vi "Data_Acquisition(I&O).vi"(7 "Cluster":T1={"valve1Switch"=FALSE, "valve2Switch"=FALSE, "valve3Switch"=FALSE, "valve4Switch"=TRUE, "valve5Switch"=FALSE, "valve6Switch"=TRUE} caption="簇") -> ()   [LabVIEW 2020]
uses:
  <vilib>/Platform/TimedLoop/XDataNode/XDataNode.xnode
  <vilib>/Platform/TimedLoop/XDataNode/nitl_modes.ctl
  <vilib>/Platform/TimedLoop/XDataNode/XDNodeRunTimeDep.lvlib
  <vilib>/Platform/TimedLoop/XDataNode/wakeup.ctl
  <vilib>/Platform/TimedLoop/XDataNode/timing_clust.ctl
  <vilib>/rvi/interface/nirviOpenFPGA/nirviOpenFPGA.xnode
  <vilib>/rvi/interface/nirviReadWriteControl/nirviReadWriteControl.xnode
  <vilib>/rvi/interface/nirviMethod/nirviMethod.xnode
  <vilib>/FPGAPlugInAG/Dynamic/niLvFpga_Download_Dynamic.vi
  <vilib>/FPGAPlugInAG/Dynamic/niLvFpga_Reset_Dynamic.vi
  <vilib>/FPGAPlugInAG/Dynamic/niLvFpga_Run_Dynamic.vi
  <vilib>/rvi/interface/nirviCloseFPGA/nirviCloseFPGA.xnode
  <vilib>/rvi/interface/Simulation/niFpgaSimulationCallBeginRW.vi
  <vilib>/rvi/errors/niLvFpgaAdjustHostInterfaceError.vi
  <vilib>/Utility/error.llb/Error Cluster From Error Code.vi
  NiFpgaLv.dll
  <vilib>/FPGAPlugInAG/Dynamic/niLvFpga_Close_Dynamic.vi
  FPGA_Link.vi
  <vilib>/FPGAPlugInAG/cRIO-9047/niLvFpga_Open_cRIO-9047.vi
  <vilib>/rvi/interface/common/dynamic/niFpgaDynamicAddResources.vi
panel:
  out "流量":dbl=0.0003509521484375
  out "泵1出口压力":dbl=0.15506744384765625
  out "泵2进口压力":dbl=0.16880035400390625
  out "Distance":dbl=0.16645648193359375
  out "P1":dbl(graph)=-16.34526252746582
  out "P2":dbl(graph)=-14.681816101074219
  out "P3":dbl(graph)=-14.679431915283203
  out "Swing_Joint_Pi":fxp<+/-,24,5>
  out "Swing_Joint_Po":fxp<+/-,24,5>
  out "Boom_Joint_Pi":fxp<+/-,24,5>
  out "Boom_Joint_Po":fxp<+/-,24,5>
  out "Stick_Joint_Pi":fxp<+/-,48,10>
  out "Stick_Joint_Po":fxp<+/-,24,5>
  out "Reference_Pressure":fxp<+/-,24,5>
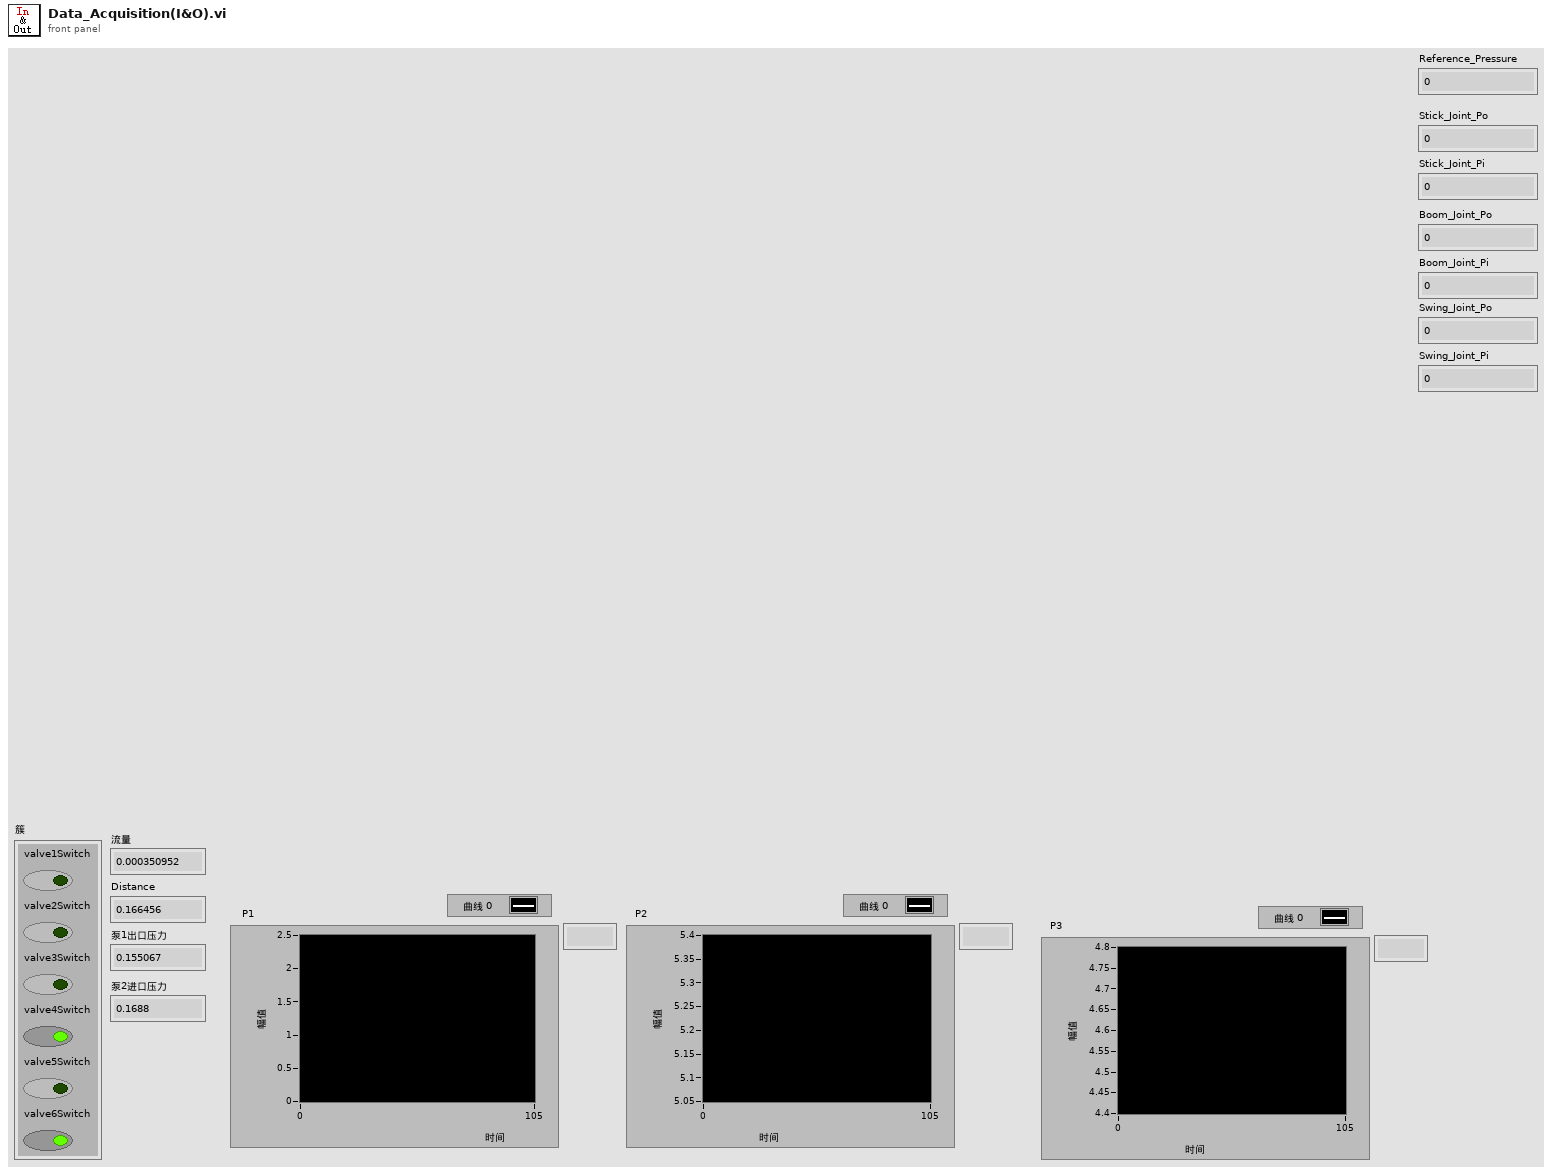
[diagram p1: front panel]
types:
  T1 = cluster{"valve1Switch":bool, "valve2Switch":bool, "valve3Switch":bool, "valve4Switch":bool, "valve5Switch":bool, "valve6Switch":bool}
  T2 = typedef "XDNodeRunTimeDep.lvlib/timing_clust.ctl" = cluster{"Expected End [f-1]":u64, "Actual End [f-1]":u64, "Finished Late? [f-1]":bool, "Expected End [i-1]":u64, "Actual End [i-1]":u64, "Finished Late? [i-1]":bool, "Expected Start [i]":u64, "Actual Start [i]":u64, "Expected Start [f]":u64, "Actual Start [f]":u64, "Source Name":string, "Structure Name":string, "Period":i64, "Deadline":i64, "Offset":i64, "Start":i64, "Priority":i32, "Timeout":i32, "Mode":T3, "Wakeup Reason":T4, "Error":errorcluster, "Source Type":string, "Secondary Source Type":string, "Global End Time":u64, "Global Start Time":u64, "Frame Duration":u64, "Iteration Duration":u64, "Assigned CPU":i32, "I/O Scan Engine Mode":u32}
  T3 = typedef "XDNodeRunTimeDep.lvlib/nitl_modes.ctl" = enum32{"No Change", "Process missed periods, maintain original phase", "Discard missed periods, maintain original phase", "Process missed periods, ignore original phase", "Discard missed periods, ignore original phase"}
  T4 = typedef "XDNodeRunTimeDep.lvlib/wakeup.ctl" = enum32{"Normal", "Aborted", "Asynchronous wakeup", "Timing source error", "Timed loop error", "Timeout"}
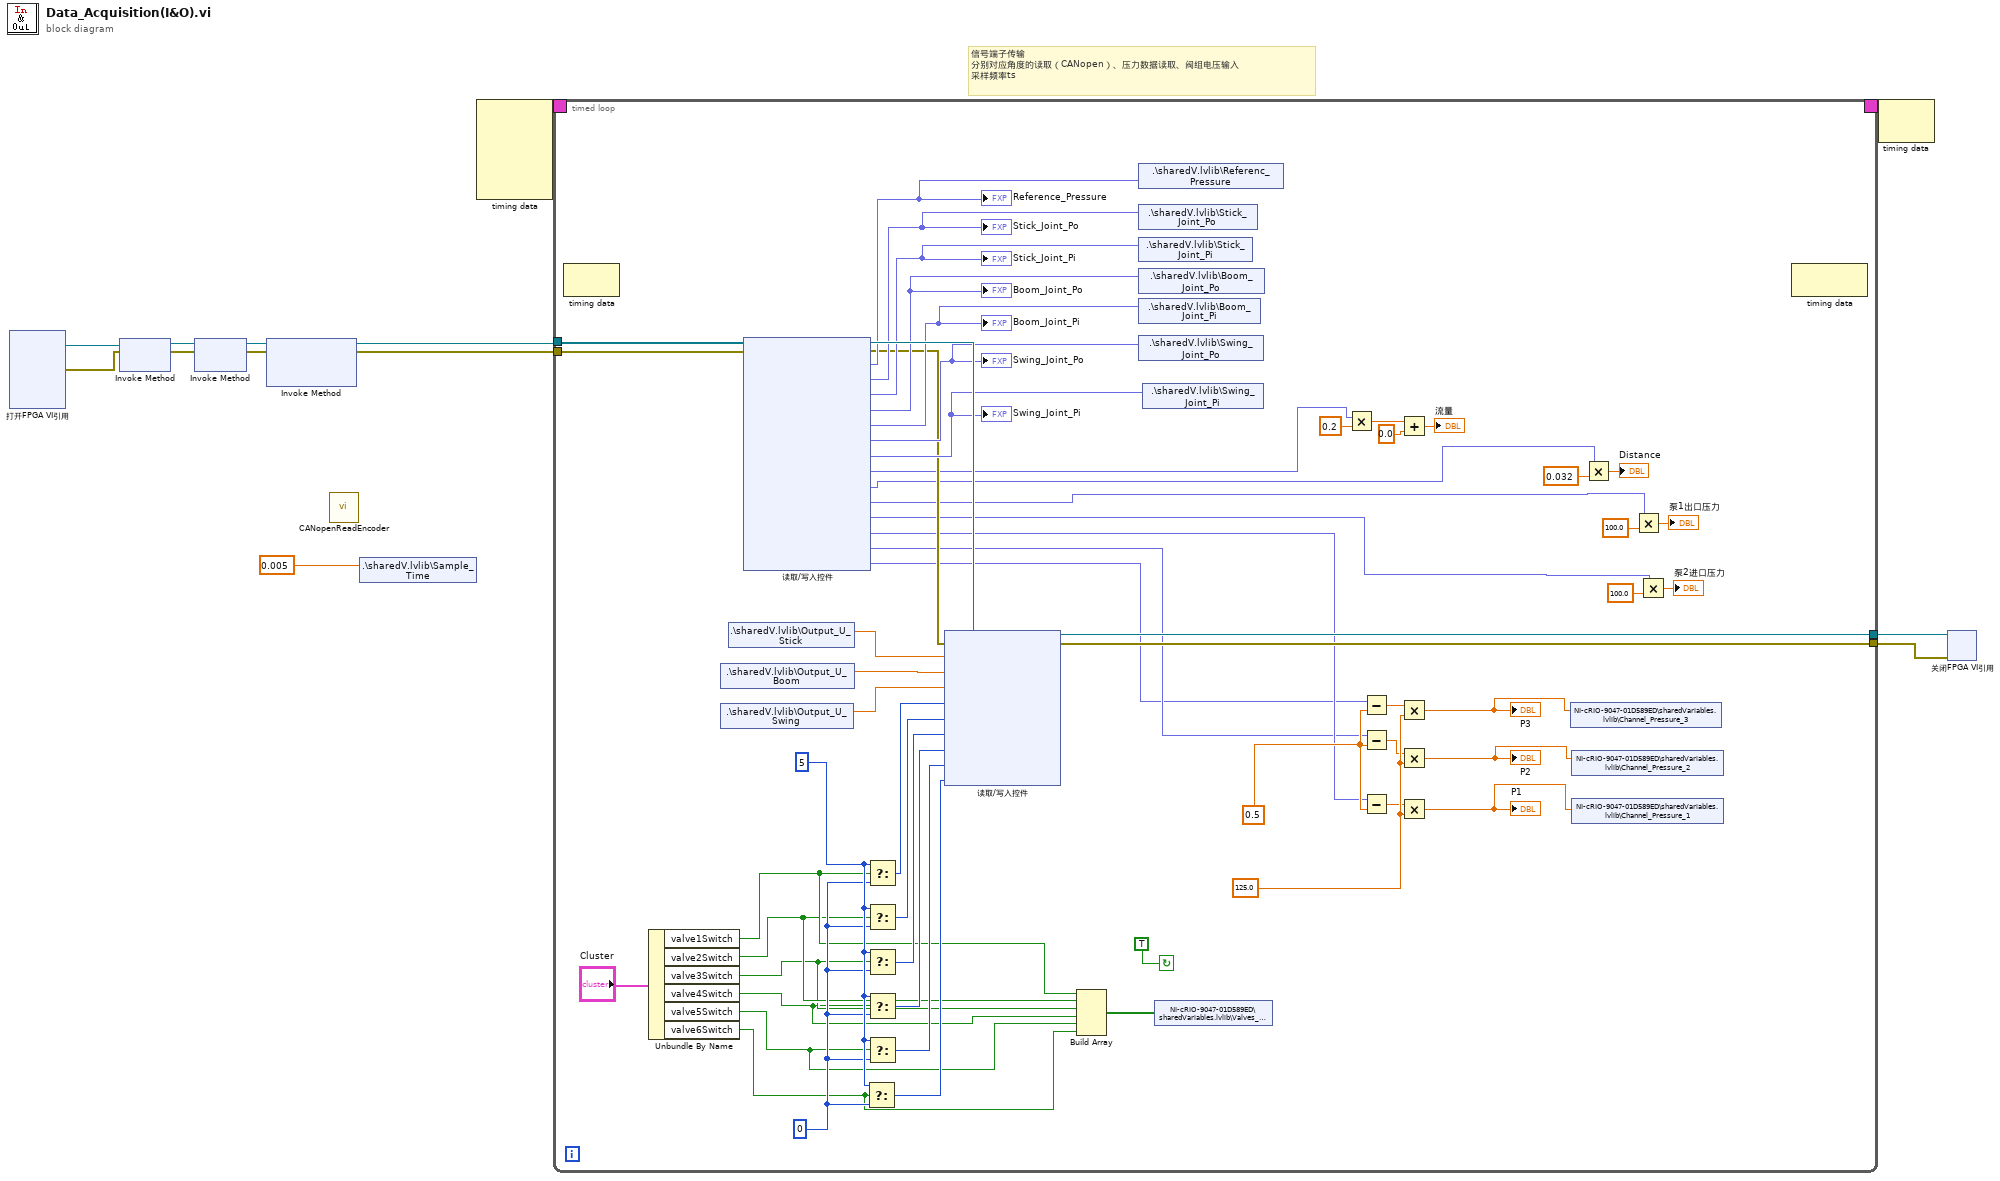
[diagram p0: block diagram]
diagram:
  # "信号端子传输\n分别对应角度的读取（CANopen）、压力数据读取、阀组电压输入\n采样频率ts"
  n1 = xnode "打开FPGA VI引用"() -> ("FPGA VI引用输出"=w4:refnum<k20>, "错误输出"=w3:errorcluster)  [unwired: 2 in]
  n2 = xnode "Invoke Method"("FPGA VI引用输入"=w4, "错误输入"=w3) -> ("FPGA VI引用输出"=w11:refnum<k20>, "错误输出"=w9:errorcluster)
  n3 = xnode "Invoke Method"("FPGA VI引用输入"=w11, "错误输入"=w9) -> ("FPGA VI引用输出"=w10:refnum<k20>, "错误输出"=w8:errorcluster)
  n4 = xnode "Invoke Method"("FPGA VI引用输入"=w10, "错误输入"=w8) -> ("FPGA VI引用输出"=w7:refnum<k20>, "错误输出"=w2:errorcluster)  [unwired: 1 in]
  n5 = call "CANopenReadEncoder.vi"() -> ()  [unwired: 3 in]
  n6 = shared-variable ".\\sharedV.lvlib\\Sample_Time"(0.005) -> ()  [unwired: 1 in, 1 out]
  n7 = node-c288() -> (w13:T2)  [unwired: 5 in]
  n8 = timed-loop {
    timing: w13 -> [_]
    timing-out: [_] -> w12
    tunnel: w7 -> [w71]
    tunnel: [w69] -> w5
    tunnel: w2 -> [w57]
    tunnel: [w55] -> w1
    stop <- TRUE continue-if-true
    w53 = 125.0
    w52 = 0.5
    w31 = 5 ("t")
    w30 = 0
    n9 = node-c288() -> ()  [unwired: 1 in, 1 out]
    n10 = Unbundle By Name("Cluster") -> ("valve1Switch"=w20:bool, "valve2Switch"=w19:bool, "valve3Switch"=w18:bool, "valve4Switch"=w17:bool, "valve5Switch"=w16:bool, "valve6Switch"=w15:bool)
    n11 = shared-variable ".\\sharedV.lvlib\\Output_U_Boom"() -> (w66:dbl)  [unwired: 1 in, 1 out]
    n12 = shared-variable ".\\sharedV.lvlib\\Output_U_Swing"() -> (w65:dbl)  [unwired: 1 in, 1 out]
    n13 = shared-variable ".\\sharedV.lvlib\\Output_U_Stick"() -> (w67:dbl)  [unwired: 1 in, 1 out]
    n14 = xnode "读取/写入控件"("FPGA VI引用输入"=w71, "错误输入"=w57) -> ("FPGA VI引用输出"=w70:refnum<k20>, "错误输出"=w56:errorcluster, "Reference_Pressure"=w64:fxp<+/-,24,5>, "Stick_Joint_Po"=w63:fxp<+/-,24,5>, "Stick_Joint_Pi"=w58:fxp<+/-,48,10>, "Boom_Joint_Po"=w59:fxp<+/-,24,5>, "Boom_Joint_Pi"=w60:fxp<+/-,24,5>, "Swing_Joint_Po"=w61:fxp<+/-,24,5>, "Swing_Joint_Pi"=w62:fxp<+/-,24,5>, "flowU"=w38:fxp<+/-,24,5>, "V_Distance"=w37:fxp<+/-,24,5>, "pump1_P"=w36:fxp<+/-,24,5>, "pump2_P"=w35:fxp<+/-,24,5>, "Chamber_P1"=w34:fxp<+/-,24,5>, "Chamber_P2"=w33:fxp<+/-,24,5>, "Chamber_P3"=w32:fxp<+/-,24,5>)
    "Reference_Pressure" <- w64
    "Stick_Joint_Po" <- w63
    "Stick_Joint_Pi" <- w58
    "Boom_Joint_Po" <- w59
    "Boom_Joint_Pi" <- w60
    "Swing_Joint_Po" <- w61
    "Swing_Joint_Pi" <- w62
    n15 = Select(t=w31, s=w15, f=w30) -> (s? t:f=w29:i32)
    n16 = Select ("选择")(t=w31, s=w20, f=w30) -> (s? t:f=w54:i32)
    n17 = Select(t=w31, s=w19, f=w30) -> (s? t:f=w28:i32)
    n18 = Select(t=w31, s=w18, f=w30) -> (s? t:f=w27:i32)
    n19 = Select(t=w31, s=w17, f=w30) -> (s? t:f=w26:i32)
    n20 = Select(t=w31, s=w16, f=w30) -> (s? t:f=w25:i32)
    n21 = xnode "读取/写入控件"("FPGA VI引用输入"=w70, "错误输入"=w56, "Stick_Joint_Input"=w67, "Boom_Joint_Input"=w66, "Swing_Joint_Input"=w65, "valve1Switch"=w54, "valve2Switch"=w28, "valve3Switch"=w27, "valve4Switch"=w26, "valve5Switch"=w25, "valve6Switch"=w29) -> ("FPGA VI引用输出"=w69:refnum<k20>, "错误输出"=w55:errorcluster)
    n22 = Build Array(w20, w19, w18, w17, w16, w15) -> (w14:bool[])
    n23 = shared-variable ".\\sharedV.lvlib\\Referenc_Pressure"(w64) -> ()  [unwired: 1 in, 1 out]
    n24 = shared-variable ".\\sharedV.lvlib\\Stick_Joint_Po"(w63) -> ()  [unwired: 1 in, 1 out]
    n25 = shared-variable ".\\sharedV.lvlib\\Stick_Joint_Pi"(w58) -> ()  [unwired: 1 in, 1 out]
    n26 = shared-variable ".\\sharedV.lvlib\\Boom_Joint_Po"(w59) -> ()  [unwired: 1 in, 1 out]
    n27 = shared-variable ".\\sharedV.lvlib\\Boom_Joint_Pi"(w60) -> ()  [unwired: 1 in, 1 out]
    n28 = shared-variable ".\\sharedV.lvlib\\Swing_Joint_Po"(w61) -> ()  [unwired: 1 in, 1 out]
    n29 = shared-variable ".\\sharedV.lvlib\\Swing_Joint_Pi"(w62) -> ()  [unwired: 1 in, 1 out]
    n30 = shared-variable "NI-cRIO-9047-01D589ED\\sharedVariables.lvlib\\Valves_Switch"(w14) -> ()  [unwired: 1 in, 1 out]
    n31 = Multiply(x=w38, y=0.2) -> (x*y=w40:dbl)
    n32 = Subtract(x=w32, y=w52) -> (x-y=w51:dbl)
    n33 = Subtract(x=w33, y=w52) -> (x-y=w50:dbl)
    n34 = Subtract(x=w34, y=w52) -> (x-y=w49:dbl)
    n35 = Add(x=w40, y=0.0) -> (x+y=→"流量":dbl)
    n36 = Multiply(x=w51, y=w53) -> (x*y=w24:dbl)
    "P3" <- w24
    n37 = Multiply(x=w50, y=w53) -> (x*y=w23:dbl)
    "P2" <- w23
    n38 = Multiply(x=w49, y=w53) -> (x*y=w22:dbl)
    "P1" <- w22
    n39 = shared-variable "NI-cRIO-9047-01D589ED\\sharedVariables.lvlib\\Channel_Pressure_3"(w24) -> ()  [unwired: 1 in, 1 out]
    n40 = shared-variable "NI-cRIO-9047-01D589ED\\sharedVariables.lvlib\\Channel_Pressure_2"(w23) -> ()  [unwired: 1 in, 1 out]
    n41 = shared-variable "NI-cRIO-9047-01D589ED\\sharedVariables.lvlib\\Channel_Pressure_1"(w22) -> ()  [unwired: 1 in, 1 out]
    n42 = Multiply(x=w37, y=0.032) -> (x*y=→"Distance":dbl)
    n43 = Multiply(x=w36, y=100.0) -> (x*y=→"泵1出口压力":dbl)
    n44 = Multiply(x=w35, y=100.0) -> (x*y=→"泵2进口压力":dbl)
    n45 = node-c288() -> ()  [unwired: 1 in, 1 out]
  }
  n46 = node-c288(w12) -> ()  [unwired: 1 out]
  n47 = xnode "关闭FPGA VI引用"("FPGA VI引用输入"=w5, "错误输入"=w1) -> ()  [unwired: 1 out]
